vi "set memory.vi"(8 "error in (no error)":errorcluster caption="에러 입력(에러 없음)", 10 "WF List":T1[](array[typedef]), 11 "DW7912 입력":refnum<class "DW7912.lvclass">) -> (0 "error out":errorcluster caption="에러 출력", 3 "DW7912 출력":refnum<class "DW7912.lvclass">)   [LabVIEW 2020, in "DW7912.lvclass"]
uses:
  DW7912.lvclass
  SubVIs/Waveform Editor/Controls/(Ctrl)Waveform Editor_WF List.ctl
  Waveform Obj Class/Waveform Obj/Waveform Obj.lvclass
  Haptic IC/Haptic IC.lvclass/Haptic IC.ctl
  SubVIs/I2C/Instance VIs/(SubVI)I2C_8Bit-8Bit_Read_Single.vi
  SubVIs/I2C/Instance VIs/(SubVI)I2C_8Bit-8Bit_Write_Single.vi
  SubVIs/I2C/Instance VIs/(SubVI)I2C_8Bit-8Bit_Write_Sequential.vi
  DW7912.lvclass/DW7912.ctl
  Haptic IC/Haptic IC.lvclass
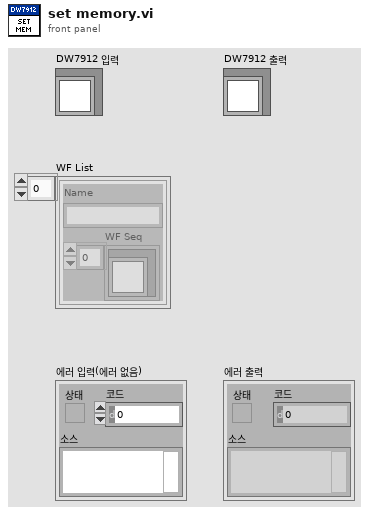
[diagram p1: front panel]
types:
  T1 = typedef "(Ctrl)Waveform Editor_WF List.ctl" = cluster{"Name":string, "WF Seq":refnum<class "Waveform Obj.lvclass">[]}
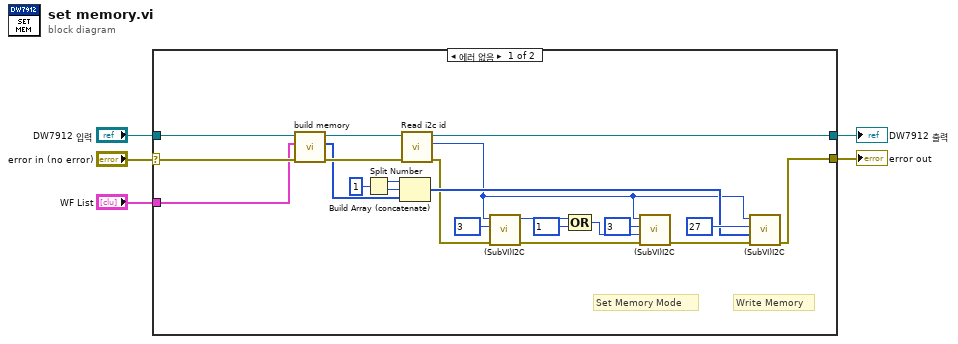
[diagram p0: block diagram]
diagram:
  n1 = case shown="에러 없음" "error in (no error)" {
    selector: "error in (no error)" -> [w20 w29]
    tunnel: [w21 w29] -> w4
    tunnel: "DW7912 입력" -> [w18 w28]
    tunnel: [w27 w28] -> w2
    tunnel: "WF List" -> [w16 _]
    frame No Error {
      # "Write Memory"
      # "Set Memory Mode"
      n2 = call-dynamic "build memory.vi"("error in (no error)"=w20, "WF List"=w16, "DW7912 입력"=w18) -> ("error out"=w19:errorcluster, "full memory data"=w15:u8[], "DW7912 출력"=w17:refnum<class "DW7912.lvclass">)  [unwired: 5 in, 1 out]
      n3 = Split Number(x=u16 1) -> (hi(x)=w24:u8, lo(x)=w23:u8)
      n4 = Build Array (concatenate)(w24, w23, w15) -> (w22:u8[])
      n5 = call "Read i2c id.vi"("error in (no error)"=w19, "Haptic IC 입력"=w17) -> ("error out"=w7:errorcluster, "i2c id"=w6:u8, "Haptic IC 출력"=w27:refnum<class "DW7912.lvclass">)  [unwired: 7 in]
      n6 = call-poly "(SubVI)I2C.vi"("error in (no error)"=w7, "Address"=u8 3, "ID"=w6) -> ("error out"=w13:errorcluster, "Read Data"=w14:u8)  [unwired: 6 in, 1 out]
      n7 = Compound Arithmetic op=OR(w14, u8 1 ("y")) -> (w12:u8)
      n8 = call-poly "(SubVI)I2C.vi"("error in (no error)"=w13, "Data to Write"=w12, "Address"=u8 3, "ID"=w6) -> ("error out"=w8:errorcluster)  [unwired: 6 in, 1 out]
      n9 = call-poly "(SubVI)I2C.vi"("error in (no error)"=w8, "Data to Write"=w22, "Start Address"=u8 27, "ID"=w6) -> ("error out"=w21:errorcluster)  [unwired: 6 in, 1 out]
    }
    frame Error {
    }
  }
  "error out" <- w4
  "DW7912 출력" <- w2
